vi "Macro#CMDExecute.vi"(3 "ProgramRef":refnum<vi>, 4 "Command":string[](array[string]), 5 "ThreadsQueue":refnum<queue>[](array[refnum]), 6 "ThreadNo.":u32, 7 "ThreadModReceive":refnum<queue>[](array[refnum]), 8 "StackIn":cluster{"Program":i32, "Prog Index":i32}[](array[cluster]), 9 "ThreadInfoIn":T1) -> (0 "StackOut":cluster{"Program":i32, "Prog Index":i32}[](array[cluster]), 1 "ThreadInfoOut":T1, 2 "ErrorCode":string)   [LabVIEW 2020]
uses:
  MainFrame/Global.vi
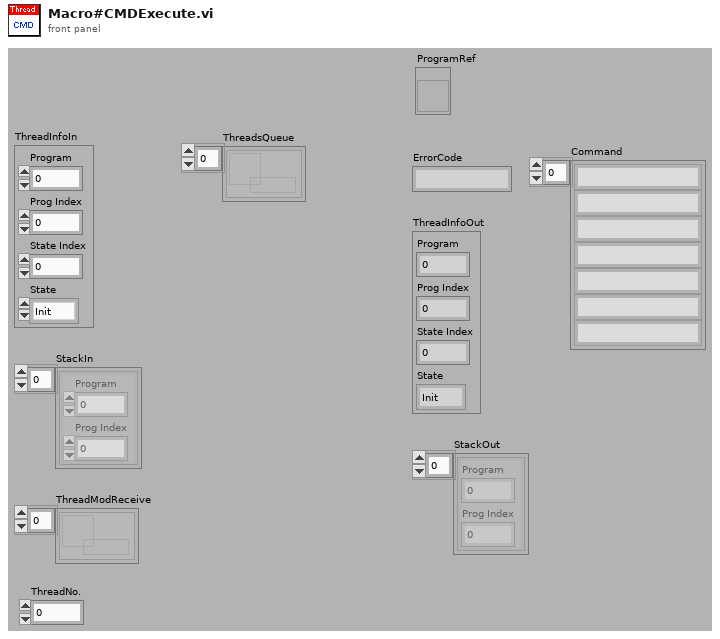
[diagram p1: front panel]
types:
  T1 = cluster{"Program":i32, "Prog Index":i32, "State Index":i32, "State":enum16{"Init", "Idle", "Auto Start", "Auto Running", "Step Start", "Step Running", "Suspend", "Restart", "Stop", "Reset"}}
  T2 = cluster{"指令":string, "代碼":string, "參數長度":i32, "乘數":dbl, "加數":dbl}[]
  T3 = enum16{"Init", "Idle", "Auto Start", "Auto Running", "Step Start", "Step Running", "Suspend", "Restart", "Stop", "Reset"}
  T4 = cluster{"指令":string, "代碼":string, "參數長度":i32, "乘數":dbl, "加數":dbl}[][]
  T5 = cluster{"指令":string, "代碼":string, "參數長度":i32, "乘數":dbl, "加數":dbl}
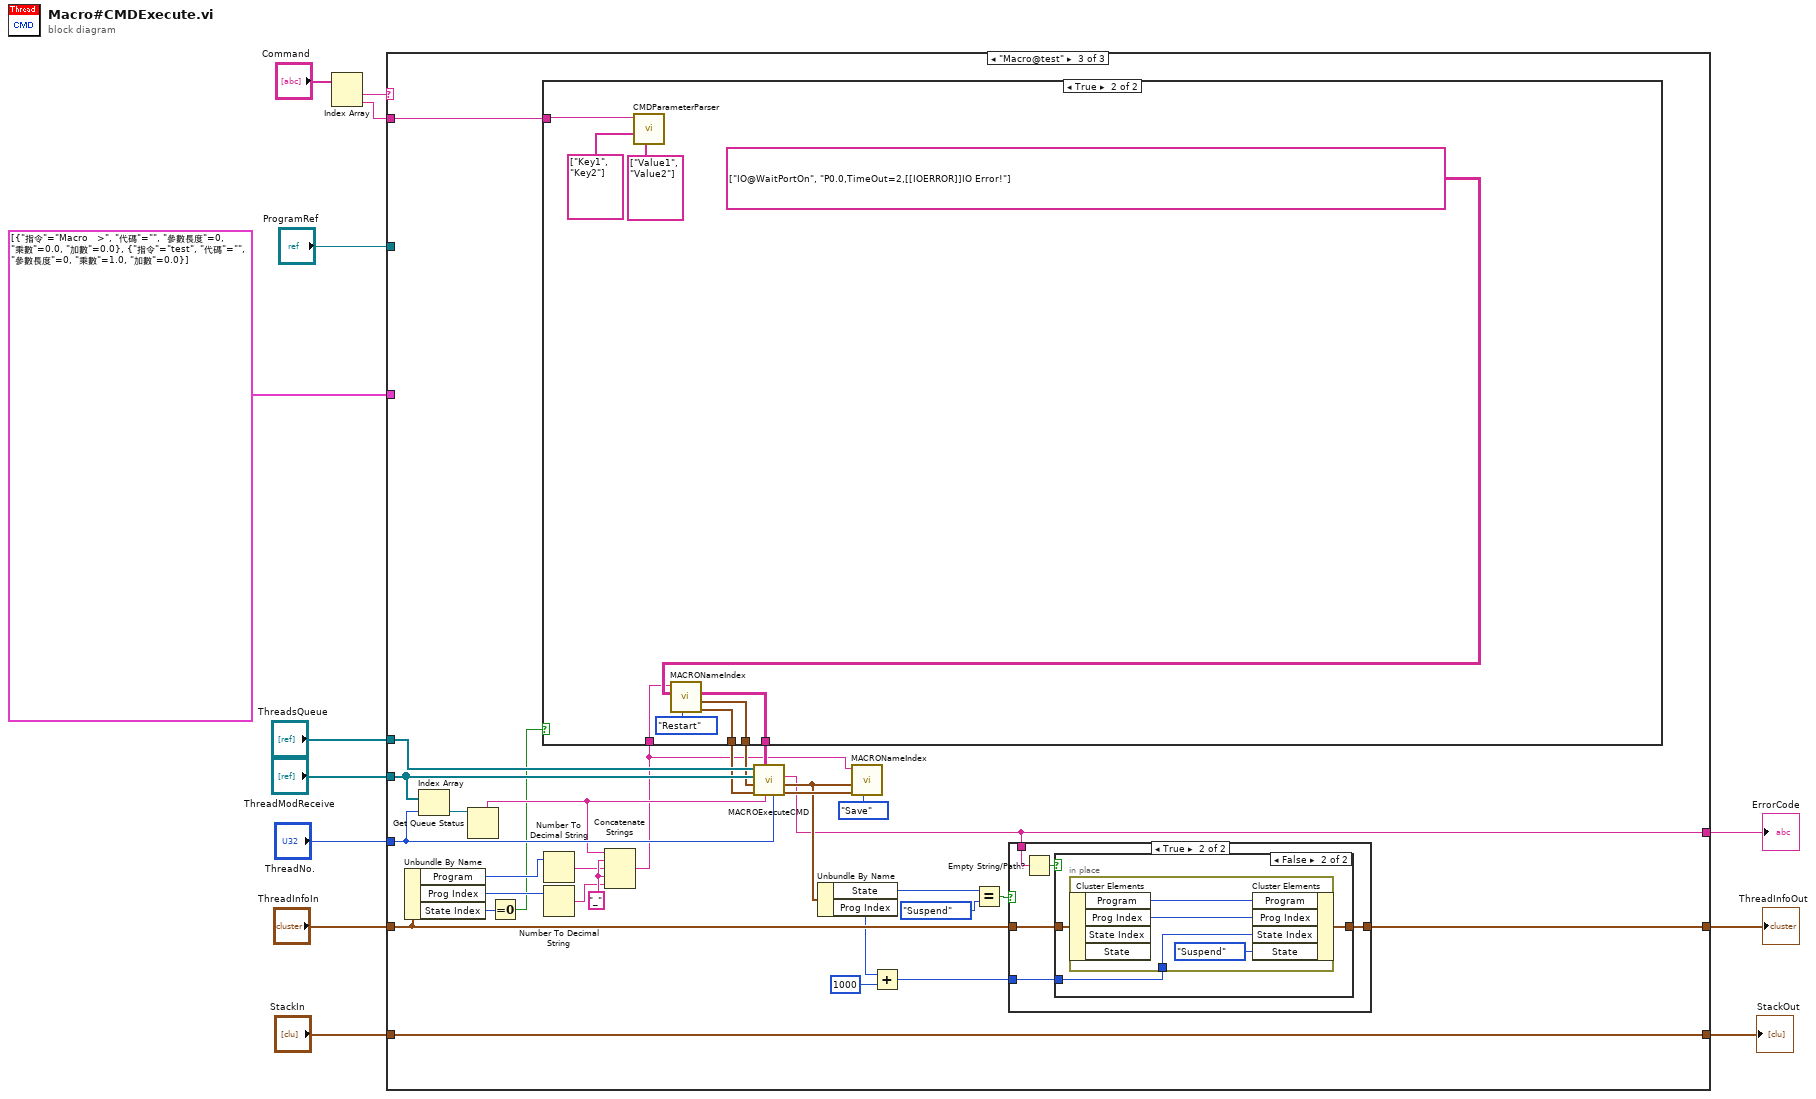
[diagram p0: block diagram]
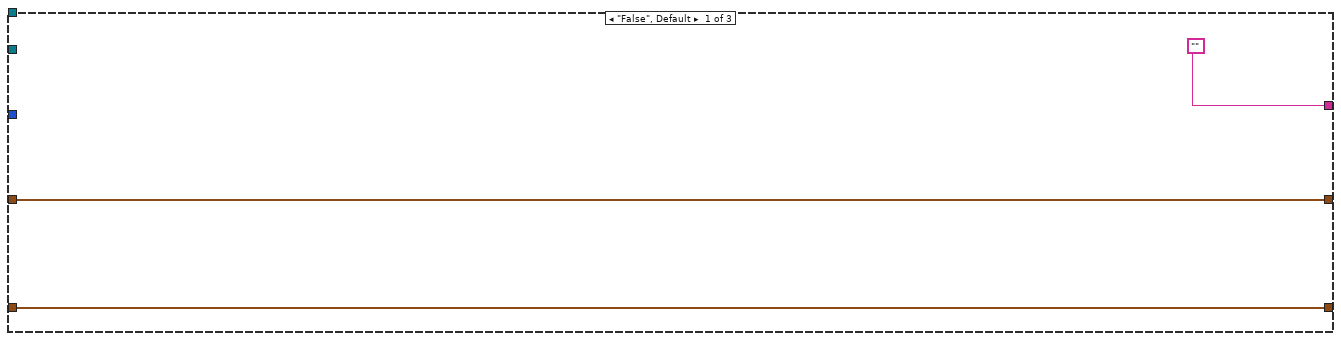
[diagram p2: hidden frame]
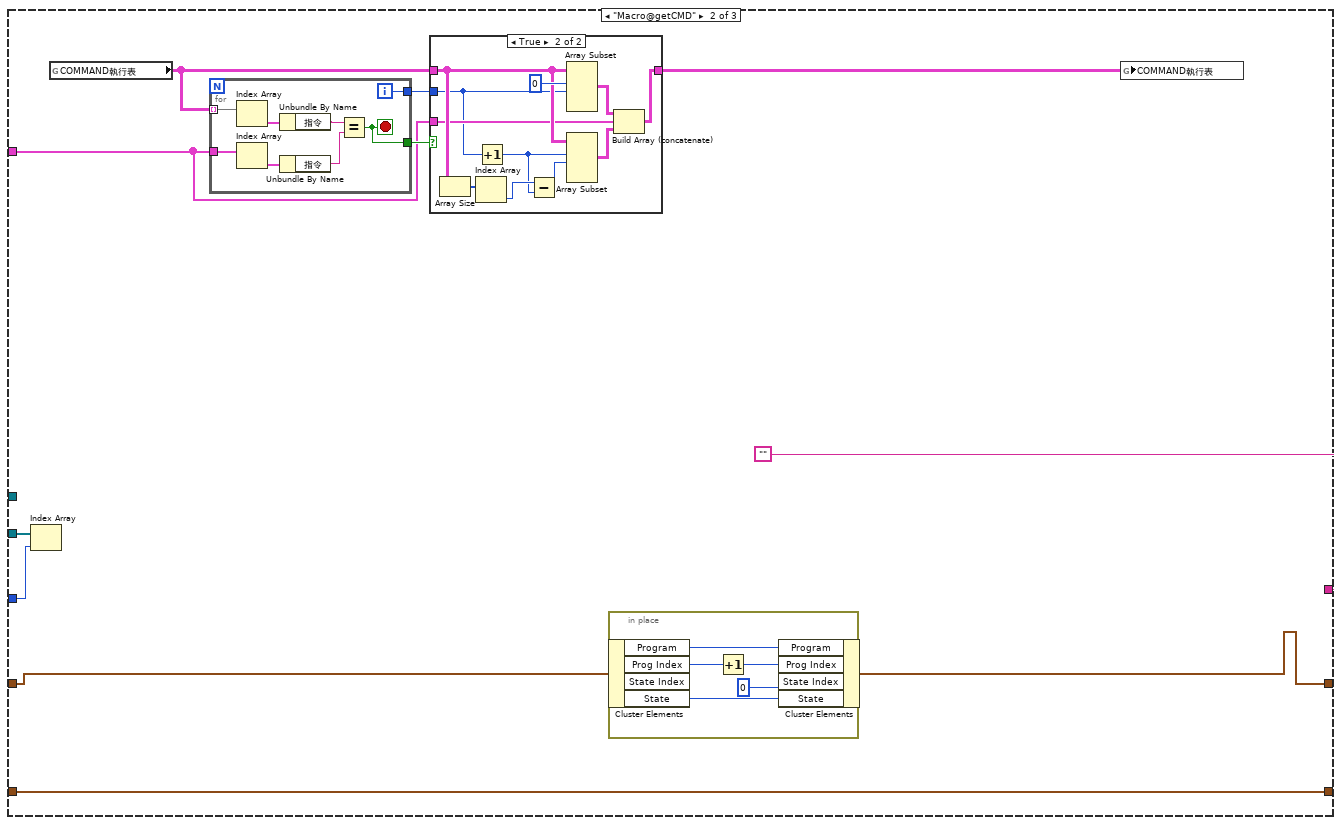
[diagram p3: hidden frame]
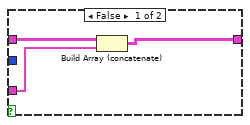
[diagram p4: hidden frame]
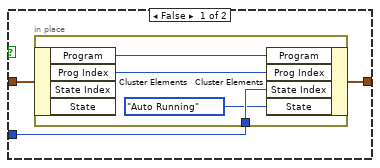
[diagram p5: hidden frame]
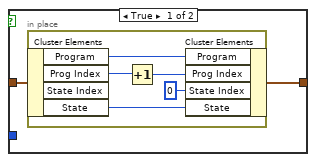
[diagram p6: hidden frame]
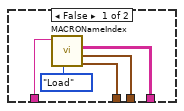
[diagram p7: hidden frame]
diagram:
  n1 = Index Array(array="Command") -> (element #1=w1:string, element #2=w9:string)  [unwired: 2 in]
  n2 = case shown="\"Macro@test\"" w1 {
    tunnel: "ThreadModReceive" -> [_ w27 w66]
    tunnel: [w16 w25 w68] -> w6
    tunnel: "ThreadInfoIn" -> [w16 w24 w69]
    tunnel: "ThreadNo." -> [_ w26 w65]
    tunnel: w9 -> [_ _ w83]
    tunnel: "ThreadsQueue" -> [_ _ w67]
    tunnel: ["" "" w55] -> w11
    tunnel: [w14 w23 w84] -> w12
    tunnel: "StackIn" -> [w14 w23 w84]
    tunnel: T2 [{"指令"="Macro   >", "代碼"="", "參數長度"=0, "乘數"=0.0, "加數"=0.0}, {"指令"="test", "代碼"="", "參數長度"=0, "乘數"=1.0, "加數"=0.0}] ("Test程式表") -> [_ w19 _]
    tunnel: "ProgramRef" -> [_ _ _]
    frame "False", Default {
    }
    frame "Macro@getCMD" {
      n3 = Index Array(array=w27, index=w26) -> ()  [unwired: 1 out]
      n4 = global read "Global.vi" "COMMAND執行表"() -> (w18:T4)
      n5 = for {
        tunnel: w18 -> [w47] mode=indexing
        tunnel: w19 -> [w48]
        tunnel: [w43] -> w20
        tunnel: [w42] -> w21
        i -> [w43]
        stop <- w42 stop-if-true
        n6 = Index Array(array=w47) -> (element=w49:T5)  [unwired: 1 in]
        n7 = Index Array(array=w48) -> (element=w46:T5)  [unwired: 1 in]
        n8 = Unbundle By Name(w49) -> ("指令"=w45:string)
        n9 = Unbundle By Name(w46) -> ("指令"=w44:string)
        n10 = Equal?(x=w45, y=w44) -> (x = y?=w42:bool)
      }
      n11 = case shown="True" w21 {
        tunnel: w20 -> [_ w32]
        tunnel: w19 -> [w29 w35]
        tunnel: w18 -> [w30 w40]
        tunnel: [w28 w33] -> w17
        frame False {
          n12 = Build Array (concatenate)(w30, w29) -> (w28:T4)
        }
        frame True {
          n13 = Array Size(array=w40) -> (size(s)=w39:i32[])
          n14 = Index Array(array=w39) -> (element=w38:i32)  [unwired: 1 in]
          n15 = Increment(x=w32) -> (x+1=w31:i32)
          n16 = Subtract(x=w38, y=w31) -> (x-y=w37:i32)
          n17 = Array Subset(array=w40, index (row)=0 ("index"), length (row)=w32) -> (w36:T4)  [unwired: 2 in]
          n18 = Array Subset(array=w40, index (row)=w31, length (row)=w37) -> (w34:T4)  [unwired: 2 in]
          n19 = Build Array (concatenate)(w36, w35, w34) -> (w33:T4)
        }
      }
      n20 = in-place {
        n21 = in-place-cluster #1(w24) -> ("Program"=w54:i32, "Prog Index"=w52:i32, "State"=w50:T3)  [unwired: 1 out]
        n22 = Increment(x=w52) -> (x+1=w53:i32)
        n23 = in-place-cluster #1("Program"=w54, "Prog Index"=w53, "State Index"=0, "State"=w50) -> (w25:T1)
      }
      n24 = global write "Global.vi" "COMMAND執行表"(w17) -> ()
    }
    frame "Macro@test" {
      w78 = "_" ("string")
      n25 = Unbundle By Name(w69) -> ("Program"=w80:i32, "Prog Index"=w79:i32, "State Index"=w81:i32)
      n26 = Index Array(array=w66, index=w65) -> (element=w82:refnum<queue>)
      n27 = Get Queue Status(queue=w82) -> (queue name=w64:string)  [unwired: 2 in, 7 out]
      n28 = Equal To 0?(x=w81) -> (x = 0?=w56:bool)
      n29 = Number To Decimal String(number=w80) -> (decimal integer string=w77:string)  [unwired: 1 in]
      n30 = Number To Decimal String(number=w79) -> (decimal integer string=w76:string)  [unwired: 1 in]
      n31 = Concatenate Strings(w64, w78, w77, w78, w76) -> (w60:string)
      n32 = case shown="True" w56 {
        tunnel: w83 -> [_ w124]
        tunnel: [w114 w119] -> w63
        tunnel: [w113 w120] -> w62
        tunnel: [w112 w118] -> w61
        tunnel: w60 -> [w111 w116]
        frame False {
          n33 = call "MACRONameIndex.vi"("OP"=enum16{"Init", "Restart", "Load", "Save"}."Load", "ID"=w111) -> ("StackOut"=w114:cluster{"Program":i32, "Prog Index":i32}[], "ThreadInfoOut"=w113:T1, "ProgramOut"=w112:string[][])  [unwired: 7 in]
        }
        frame True {
          n34 = call "CMDParameterParser.vi"("DeafultValues"=string[] ["Value1", "Value2"] ("RequiredKeys"), "RequiredKeys"=string[] ["Key1", "Key2"], "CMDParameter"=w124) -> ()  [unwired: 6 in, 3 out]
          n35 = call "MACRONameIndex.vi"("OP"=enum16{"Init", "Restart", "Load", "Save"}."Restart", "Program"=string[][] [["IO@WaitPortOn", "P0.0,TimeOut=2,[[IOERROR]]IO Error!"]], "ID"=w116) -> ("StackOut"=w119:cluster{"Program":i32, "Prog Index":i32}[], "ThreadInfoOut"=w120:T1, "ProgramOut"=w118:string[][])  [unwired: 6 in]
        }
      }
      n36 = call "MACROExecuteCMD.vi"("ThreadNo"=w65, "ProgramSelect"=w64, "MacroProgram"=w61, "StackIn"=w63, "ThreadInfoIn"=w62, "Thread Mod ReciveS"=w66, "Threads"=w67) -> ("StackOut"=w74:cluster{"Program":i32, "Prog Index":i32}[], "ThreadInfoOut"=w73:T1, "ErrorOut"=w55:string)  [unwired: 2 in]
      n37 = Unbundle By Name(w73) -> ("State"=w72:T3, "Prog Index"=w58:i32)
      n38 = call "MACRONameIndex.vi"("OP"=enum16{"Init", "Restart", "Load", "Save"}."Save", "StackIn"=w74, "ThreadInfoIn"=w73, "ID"=w60) -> ()  [unwired: 5 in, 3 out]
      n39 = Add(x=w58, y=1000) -> (x+y=w59:i32)
      n40 = Equal?(x=w72, y=T3."Suspend") -> (x = y?=w70:bool)
      n41 = case shown="True" w70 {
        tunnel: w69 -> [w87 w96]
        tunnel: [w86 w95] -> w68
        tunnel: w59 -> [w85 w92]
        tunnel: w55 -> [_ w93]
        frame False {
          n42 = in-place {
            in-place-border: w85 -> [w89]
            n43 = in-place-cluster #2(w87) -> ("Program"=w91:i32, "Prog Index"=w90:i32)  [unwired: 2 out]
            n44 = in-place-cluster #2("Program"=w91, "Prog Index"=w90, "State Index"=w89, "State"=T3."Auto Running") -> (w86:T1)
          }
        }
        frame True {
          n45 = Empty String/Path?(string/path=w93) -> (empty?=w94:bool)
          n46 = case shown="False" w94 {
            tunnel: w96 -> [w98 w106]
            tunnel: [w97 w105] -> w95
            tunnel: w92 -> [_ w104]
            frame True {
              n47 = in-place {
                n48 = in-place-cluster #3(w98) -> ("Program"=w103:i32, "Prog Index"=w102:i32, "State"=w99:T3)  [unwired: 1 out]
                n49 = Increment(x=w102) -> (x+1=w101:i32)
                n50 = in-place-cluster #3("Program"=w103, "Prog Index"=w101, "State Index"=0, "State"=w99) -> (w97:T1)
              }
            }
            frame False {
              n51 = in-place {
                in-place-border: w104 -> [w107]
                n52 = in-place-cluster #4(w106) -> ("Program"=w110:i32, "Prog Index"=w109:i32)  [unwired: 2 out]
                n53 = in-place-cluster #4("Program"=w110, "Prog Index"=w109, "State Index"=w107, "State"=T3."Suspend") -> (w105:T1)
              }
            }
          }
        }
      }
    }
  }
  "StackOut" <- w12
  "ErrorCode" <- w11
  "ThreadInfoOut" <- w6
